vi "ReadCount.vi"(11 "TypedCircularBuffer in":refnum<class "RotateCircularBuffer.lvclass">) -> (2 "size":u32, 3 "TypedCircularBuffer out":refnum<class "RotateCircularBuffer.lvclass">)   [LabVIEW 2024, in "RotateCircularBuffer.lvclass"]
uses:
  RotateCircularBuffer.lvclass
  RotateCircularBuffer.lvclass/RotateCircularBuffer.ctl
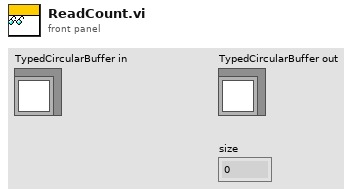
[diagram p1: front panel]
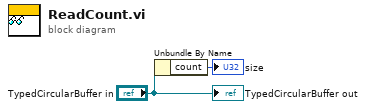
[diagram p0: block diagram]
diagram:
  n1 = Unbundle By Name("TypedCircularBuffer in") -> ("count"=→"size":u32)
  "TypedCircularBuffer out" <- "TypedCircularBuffer in"
